vi "Timer_Destroy.vi"(8 "error in (no error)":errorcluster caption="错误输入（无错误）", 11 "Timer 输入":refnum<class "Timer.lvclass">) -> (0 "error out":errorcluster caption="错误输出", 3 "Timer 输出":refnum<class "Timer.lvclass">)   [LabVIEW 2019, in "Timer.lvclass"]
uses:
  Timer.lvclass
  Timer.lvclass/Timer.ctl
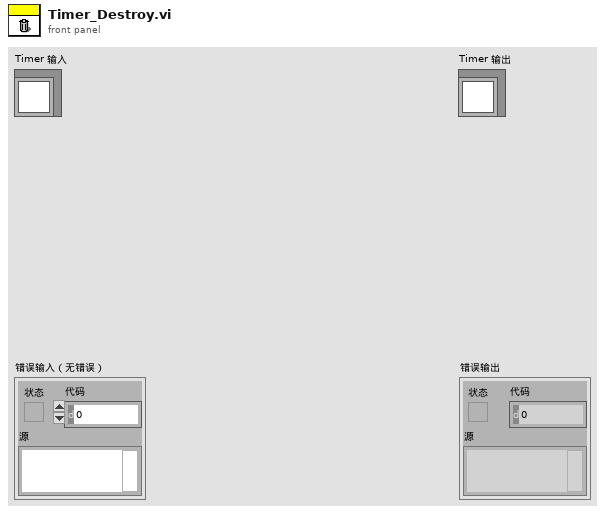
[diagram p1: front panel]
types:
  T1 = typedef "Timer.lvclass/Attribute.ctl" = cluster{"计时？":bool, "计时 (ms)":u32, "停止通知":refnum<notifier>}
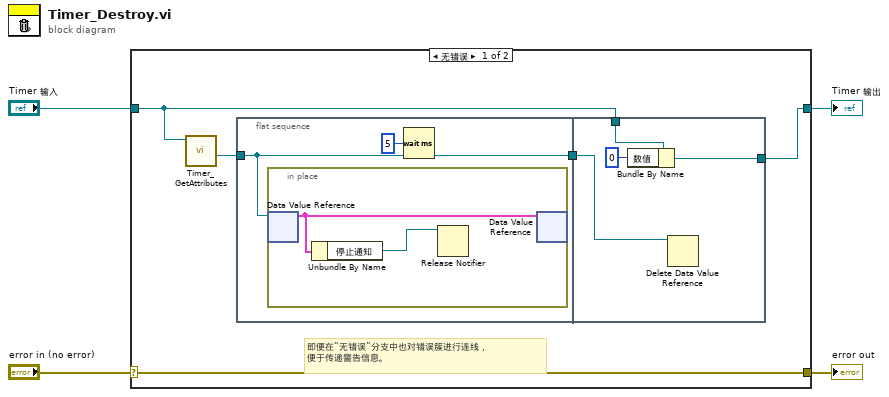
[diagram p0: block diagram]
diagram:
  n1 = case shown="无错误" "error in (no error)" {
    selector: "error in (no error)" -> [w9 w19]
    tunnel: [w9 w19] -> w3
    tunnel: [w5 w18] -> w1
    tunnel: "Timer 输入" -> [w6 w18]
    frame No Error {
      # "即便在“无错误”分支中也对错误簇进行连线，\n便于传递警告信息。"
      n2 = call "Timer_GetAttributes.vi"("Timer 输入"=w6) -> ("数据值引用"=w8:refnum<data-value>)  [unwired: 7 in, 3 out]
      n3 = flat-sequence {
        tunnel: w8 -> [w11]
        tunnel: [w11] -> w7
        tunnel: w7 -> [w17]
        tunnel: w6 -> [w16]
        tunnel: [w14] -> w5
        frame #0 {
          n4 = in-place {
            n5 = in-place-dvr #1(w11) -> (w13:T1)  [unwired: 1 out]
            n6 = Unbundle By Name(w13) -> ("停止通知"=w12:refnum<notifier>)
            n7 = Release Notifier(notifier=w12) -> ()  [unwired: 2 in, 3 out]
            n8 = in-place-dvr #1(w13) -> ()  [unwired: 2 out]
          }
          n9 = Wait (ms)(milliseconds to wait=u32 5 ("等待时间（毫秒）")) -> ()  [unwired: 1 out]
        }
        frame #1 {
          n10 = Bundle By Name(cluster=w16, "数值"=u32 0) -> (w14:refnum<class "Timer.lvclass">)
          n11 = Delete Data Value Reference(data value reference=w17) -> ()  [unwired: 1 in, 2 out]
        }
      }
    }
    frame Error {
    }
  }
  "error out" <- w3
  "Timer 输出" <- w1
